vi "S4ICS Batch Processor.vi"() -> ()   [LabVIEW 2018]
uses:
  <vilib>/addons/zeromq/socket_type.ctl
  <vilib>/addons/zeromq/socket_options.ctl
  <vilib>/addons/zeromq/zmq_context.lvclass
  <vilib>/addons/zeromq/zeromq.lvlib
  <vilib>/addons/zeromq/zmq_socket.lvclass
panel:
  out "REQ":bool
  out "SUB":bool
  in  "batch file path":path
  in  "start":bool
  out "finish":bool
  in  "S4ICS REQ endpoint":string="tcp://192.168.1.170:54883"
  out "ASEL_RDY":bool
  out "GMIR_RDY":bool
  out "GFOC_RDY":bool
  out "CALW_RDY":bool
  out "WPSEL_RDY":bool
  out "WPROT_RDY":bool
  out "S4ICS PUB DATA":string
  out "PUB":bool
  in  "S4ICS PUB endpoint":string="tcp://192.168.1.170:54880"
  out "cmd #":i32
  out "current time":timestamp format="%<%H:%M:%S%3u\n%Y/%m/%d>T"
  out "batch cmd":string
  in  "allin":T1={"s4icsIP"="localhost", "s4icsPort"=54165, "mech name"="", "cmd"=[], "log"=refnum} {"s4icsPort" min=1025 step=1}
  in  "stop":bool
  # "S4ICS ZeroMQ Monitor and Batch Command Processor"
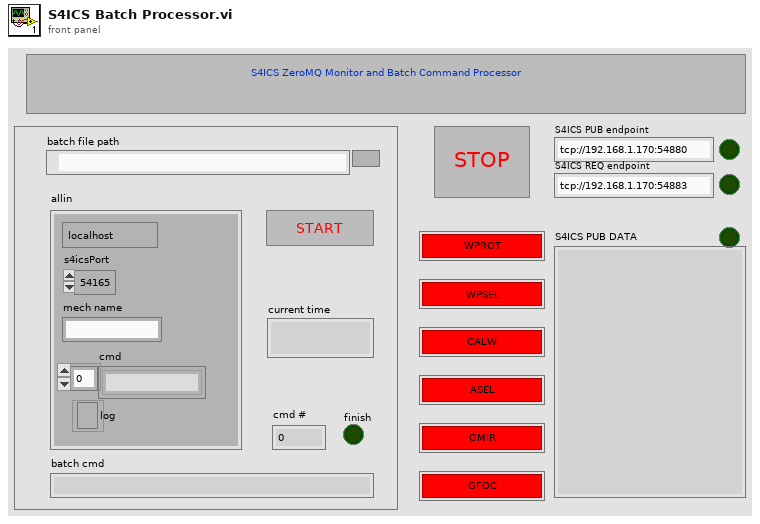
[diagram p1: front panel]
types:
  T1 = cluster{"s4icsIP":string, "s4icsPort":u16, "mech name":string, "cmd":string[], "log":refnum<file>}
  T2 = typedef "zeromq.lvlib/socket_type.ctl" = enum8{"ZMQ_PAIR", "ZMQ_PUB", "ZMQ_SUB", "ZMQ_REQ", "ZMQ_REP", "ZMQ_DEALER", "ZMQ_ROUTER", "ZMQ_PULL", "ZMQ_PUSH", "ZMQ_XPUB", "ZMQ_XSUB", "ZMQ_STREAM", "ZMQ_SERVER", "ZMQ_CLIENT", "ZMQ_RADIO", "ZMQ_DISH", "ZMQ_GATHER", "ZMQ_SCATTER", "ZMQ_DGRAM"}
  T3 = typedef "zeromq.lvlib/socket_options.ctl" = enum8{"NONE", "ZMQ_HWM", "<2>", "ZMQ_SWAP", "ZMQ_AFFINITY", "ZMQ_ROUTING_ID", "ZMQ_SUBSCRIBE", "ZMQ_UNSUBSCRIBE", "ZMQ_RATE", "ZMQ_RECOVERY_IVL", "ZMQ_MCAST_LOOP", "ZMQ_SNDBUF", "ZMQ_RCVBUF", "ZMQ_RCVMORE", "ZMQ_FD", "ZMQ_EVENTS", "ZMQ_TYPE", "ZMQ_LINGER", "ZMQ_RECONNECT_IVL", "ZMQ_BACKLOG", "ZMQ_RECOVERY_IVL_MSEC", "ZMQ_RECONNECT_IVL_MAX", "ZMQ_MAXMSGSIZE", "ZMQ_SNDHWM", "ZMQ_RCVHWM", "ZMQ_MULTICAST_HOPS", "<26>", "ZMQ_RCVTIMEO", "ZMQ_SNDTIMEO", "<29>", "<30>", "ZMQ_IPV4ONLY", "ZMQ_LAST_ENDPOINT", "ZMQ_ROUTER_MANDATORY", "ZMQ_TCP_KEEPALIVE", "ZMQ_TCP_KEEPALIVE_CNT", "ZMQ_TCP_KEEPALIVE_IDLE", "ZMQ_TCP_KEEPALIVE_INTVL", "ZMQ_TCP_ACCEPT_FILTER", "ZMQ_IMMEDIATE", "ZMQ_XPUB_VERBOSE", "ZMQ_ROUTER_RAW", "ZMQ_IPV6", "ZMQ_MECHANISM", "ZMQ_PLAIN_SERVER", "ZMQ_PLAIN_USERNAME", "ZMQ_PLAIN_PASSWORD", "ZMQ_CURVE_SERVER", "ZMQ_CURVE_PUBLICKEY", "ZMQ_CURVE_SECRETKEY", "ZMQ_CURVE_SERVERKEY", "ZMQ_PROBE_ROUTER", "ZMQ_REQ_CORRELATE", "ZMQ_REQ_RELAXED", "ZMQ_CONFLATE", "ZMQ_ZAP_DOMAIN", "ZMQ_ROUTER_HANDOVER", "ZMQ_TOS", "ZMQ_IPC_FILTER_PID", "ZMQ_IPC_FILTER_UID", "ZMQ_IPC_FILTER_GID", "ZMQ_CONNECT_ROUTING_ID", "ZMQ_GSSAPI_SERVER", "ZMQ_GSSAPI_PRINCIPAL", "ZMQ_GSSAPI_SERVICE_PRINCIPAL", "ZMQ_GSSAPI_PLAINTEXT", "ZMQ_HANDSHAKE_IVL", "<67>", "ZMQ_SOCKS_PROXY", "ZMQ_XPUB_NODROP", "ZMQ_BLOCKY", "ZMQ_XPUB_MANUAL", "ZMQ_XPUB_WELCOME_MSG", "ZMQ_STREAM_NOTIFY", "ZMQ_INVERT_MATCHING", "ZMQ_HEARTBEAT_IVL", "ZMQ_HEARTBEAT_TTL", "ZMQ_HEARTBEAT_TIMEOUT", "ZMQ_XPUB_VERBOSER", "ZMQ_CONNECT_TIMEOUT", "ZMQ_TCP_MAXRT", "ZMQ_THREAD_SAFE", "<82>", "<83>", "ZMQ_MULTICAST_MAXTPDU", "ZMQ_VMCI_BUFFER_SIZE", "ZMQ_VMCI_BUFFER_MIN_SIZE", "ZMQ_VMCI_BUFFER_MAX_SIZE", "ZMQ_VMCI_CONNECT_TIMEOUT", "ZMQ_USE_FD", "ZMQ_GSSAPI_PRINCIPAL_NAMETYPE", "ZMQ_GSSAPI_SERVICE_PRINCIPAL_NAMETYPE", "ZMQ_BINDTODEVICE", "ZMQ_ZAP_ENFORCE_DOMAIN", "ZMQ_LOOPBACK_FASTPATH", "ZMQ_METADATA", "ZMQ_MULTICAST_LOOP", "ZMQ_ROUTER_NOTIFY"}
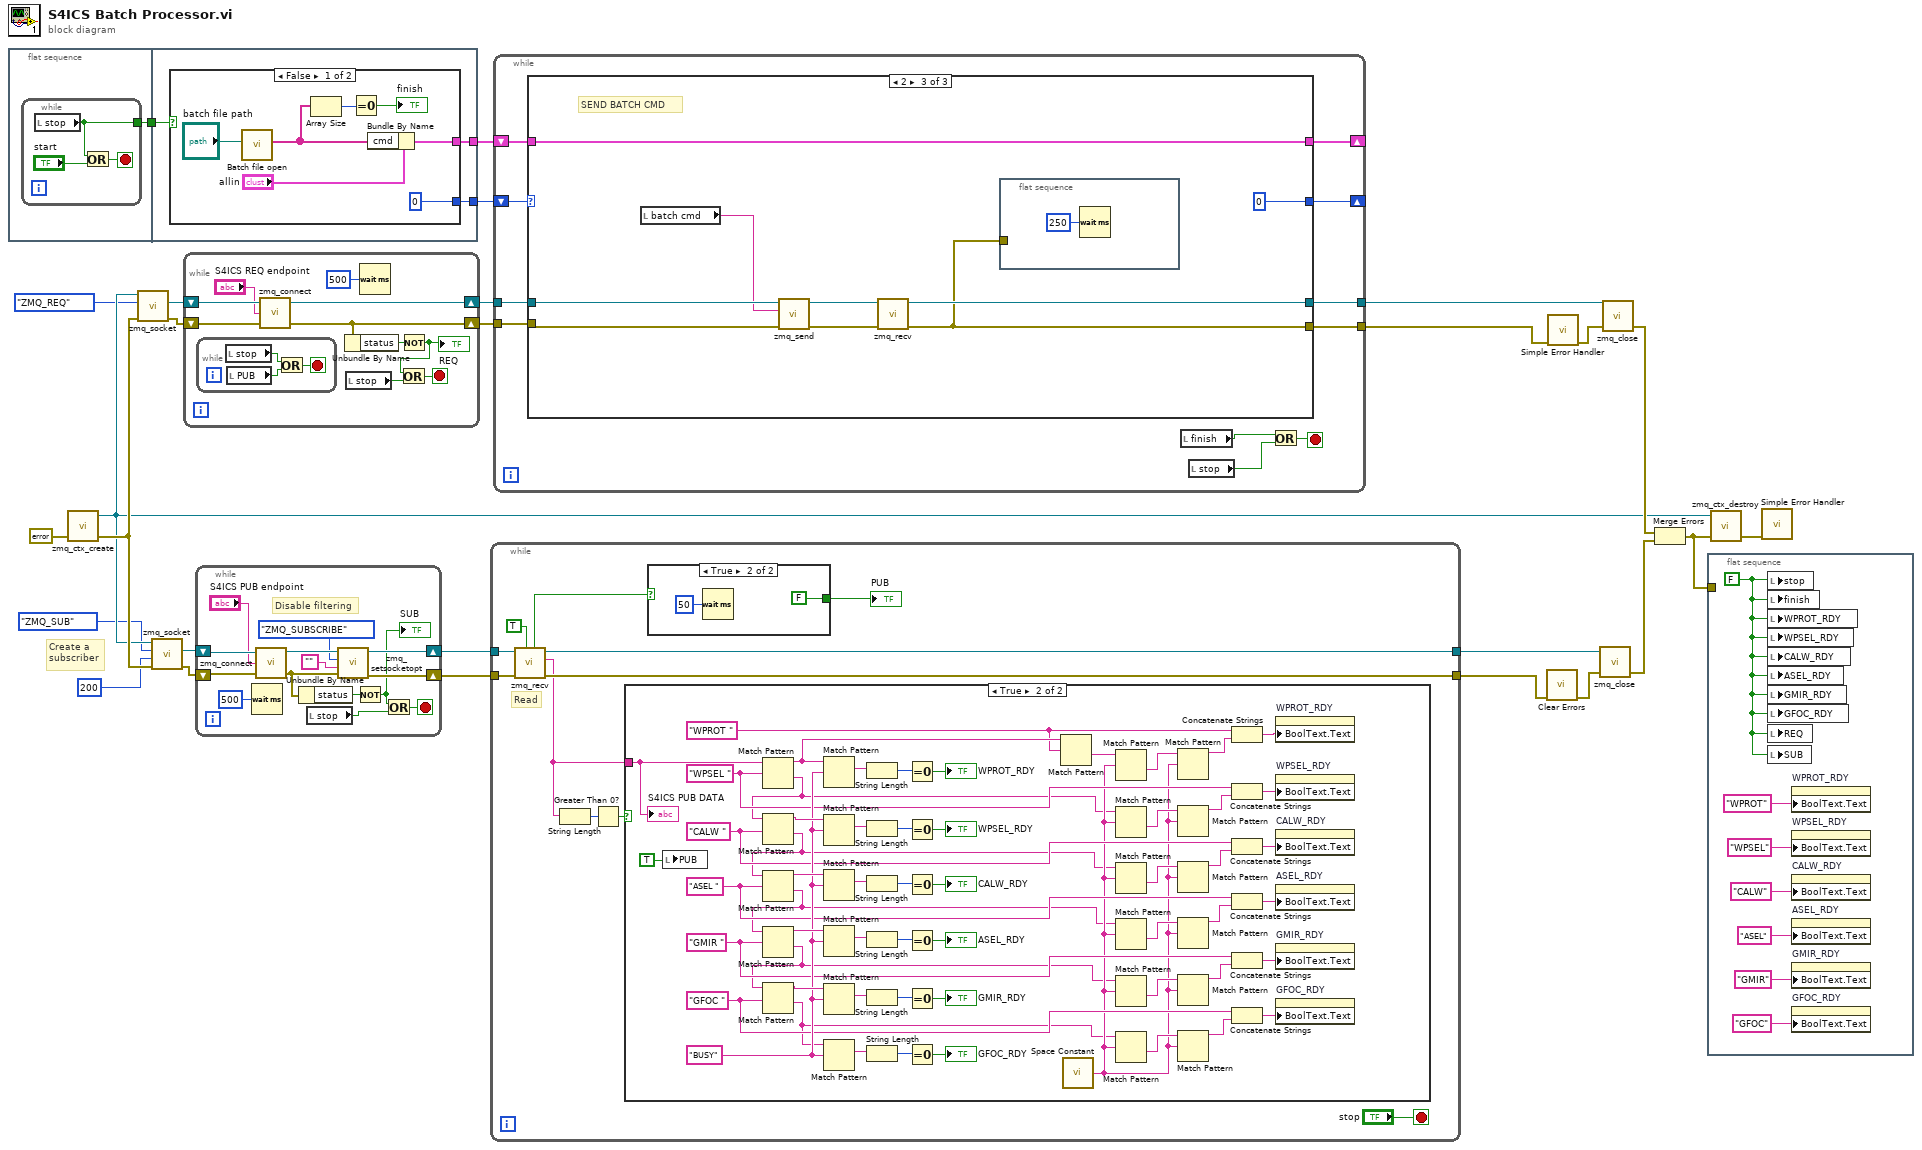
[diagram p0: block diagram]
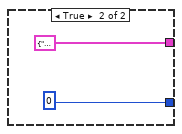
[diagram p2: hidden frame]
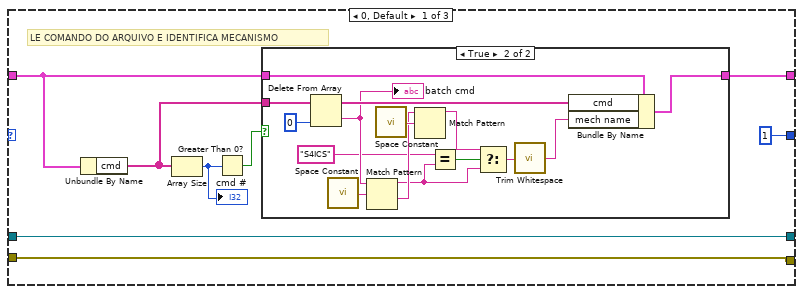
[diagram p3: hidden frame]
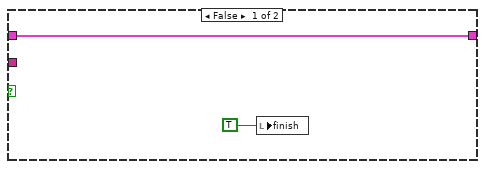
[diagram p4: hidden frame]
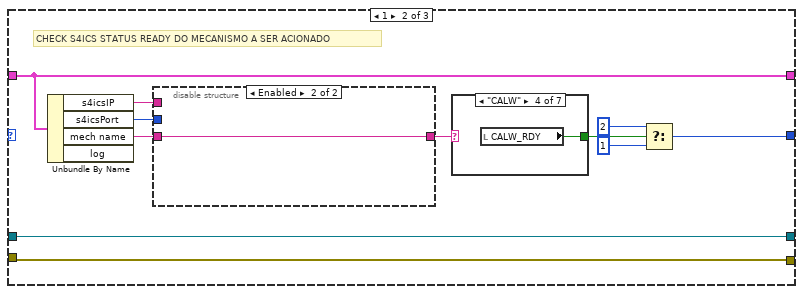
[diagram p5: hidden frame]
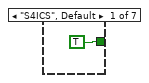
[diagram p6: hidden frame]
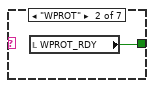
[diagram p7: hidden frame]
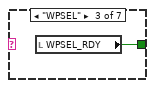
[diagram p8: hidden frame]
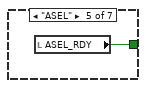
[diagram p9: hidden frame]
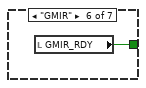
[diagram p10: hidden frame]
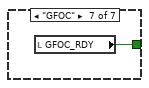
[diagram p11: hidden frame]
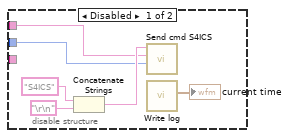
[diagram p12: hidden frame]
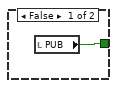
[diagram p14: hidden frame]
diagram:
  # "Create a \nsubscriber"
  n1 = flat-sequence {
    tunnel: [w28] -> w6
    tunnel: [w34] -> w16
    tunnel: [w33] -> w15
    tunnel: w6 -> [w32]
    frame #0 {
      n2 = while {
        tunnel: [w29] -> w28
        stop <- w30 stop-if-true
        n3 = local read "stop"() -> (w29:bool)
        n4 = Or(x=w29, y="start") -> (x .or. y?=w30:bool)
      }
    }
    frame #1 {
      n5 = case shown="False" w32 {
        tunnel: [u8 0 u8 0] -> w34
        tunnel: [w39 T1 {"s4icsIP"="", "s4icsPort"=0, "mech name"="", "cmd"=[], "log"=refnum} ("output cluster")] -> w33
        frame False {
          n6 = call "Batch file open.vi"("file path (use dialog)"="batch file path") -> ("cmd"=w38:string[])  [unwired: 10 in]
          n7 = Array Size(array=w38) -> (size(s)=w37:i32)
          n8 = Equal To 0?(x=w37) -> (x = 0?=→"finish":bool)
          n9 = Bundle By Name(cluster="allin", "cmd"=w38) -> (w39:T1)
        }
        frame True {
        }
      }
    }
  }
  n10 = call <vilib>:"zmq_ctx_create.vi"("error in"=errorcluster {"status"=FALSE, "code"=0, "source"=""}) -> ("error out"=w22:errorcluster, "context out"=w19:refnum<class "zmq_context.lvclass">)  [unwired: 3 in]
  n11 = call <vilib>:"zmq_socket.vi"("error in"=w22, "socket type"=socket_type."ZMQ_REQ", "context in"=w19) -> ("error out"=w14:errorcluster, "socket out"=w13:refnum<class "zmq_socket.lvclass">)  [unwired: 2 in, 1 out]
  n12 = call <vilib>:"zmq_socket.vi"("error in"=w22, "linger (ms)"=200, "socket type"=socket_type."ZMQ_SUB", "context in"=w19) -> ("error out"=w4:errorcluster, "socket out"=w3:refnum<class "zmq_socket.lvclass">)  [unwired: 1 in, 1 out]
  n13 = while {
    shift-right: [w49] -> w10
    shift-left: w14 -> [w53]
    shift-right: [w50] -> w11
    shift-left: w13 -> [w52]
    stop <- w46 stop-if-true
    n14 = while {
      stop <- w54 stop-if-true
      n15 = local read "stop"() -> (w55:bool)
      n16 = local read "PUB"() -> (w56:bool)
      n17 = Or(x=w55, y=w56) -> (x .or. y?=w54:bool)
    }
    n18 = call <vilib>:"zmq_connect.vi"("error in"=w53, "endpoint"="S4ICS REQ endpoint", "socket in"=w52) -> ("error out"=w49:errorcluster, "socket out"=w50:refnum<class "zmq_socket.lvclass">)  [unwired: 1 in]
    n19 = Unbundle By Name(w49) -> ("status"=w48:bool)
    n20 = local read "stop"() -> (w45:bool)
    n21 = Wait (ms)(milliseconds to wait=u32 500) -> ()  [unwired: 1 out]
    n22 = Not(x=w48) -> (.not. x?=w44:bool)
    "REQ" <- w44
    n23 = Or(x=w44, y=w45) -> (x .or. y?=w46:bool)
  }
  n24 = while {
    shift-right: [w70] -> w27
    shift-left: w4 -> [w68]
    shift-right: [w69] -> w26
    shift-left: w3 -> [w64]
    stop <- w59 stop-if-true
    # "Disable filtering"
    n25 = Wait (ms)(milliseconds to wait=u32 500) -> ()  [unwired: 1 out]
    n26 = call <vilib>:"zmq_connect.vi"("error in"=w68, "endpoint"="S4ICS PUB endpoint", "socket in"=w64) -> ("error out"=w60:errorcluster, "socket out"=w67:refnum<class "zmq_socket.lvclass">)  [unwired: 1 in]
    n27 = Unbundle By Name(w60) -> ("status"=w61:bool)
    n28 = local read "stop"() -> (w62:bool)
    n29 = call <vilib>:"zmq_setsocketopt.vi"("error in"=w60, "value"="", "option"=socket_options."ZMQ_SUBSCRIBE", "socket in"=w67) -> ("error out"=w70:errorcluster, "socket out"=w69:refnum<class "zmq_socket.lvclass">)  [unwired: 2 in]
    n30 = Not(x=w61) -> (.not. x?=w57:bool)
    "SUB" <- w57
    n31 = Or(x=w57, y=w62) -> (x .or. y?=w59:bool)
  }
  n32 = while {
    tunnel: w27 -> [w79]
    tunnel: w26 -> [w80]
    tunnel: [w76] -> w23
    tunnel: [w75] -> w25
    stop <- "stop" stop-if-true
    # "Read"
    n33 = call <vilib>:"zmq_recv.vi"("no block? (F)"=TRUE, "error in"=w79, "socket in"=w80) -> ("error out"=w75:errorcluster, "data"=w72:string, "socket out"=w76:refnum<class "zmq_socket.lvclass">, "timeout?"=w78:bool)  [unwired: 2 in, 1 out]
    n34 = String Length(string=w72) -> (length=w74:i32)
    n35 = Greater Than 0?(x=w74) -> (x > 0?=w73:bool)
    n36 = case shown="True" w73 {
      tunnel: w72 -> [_ w137]
      frame False {
      }
      frame True {
        w111 = "WPROT " ("regular expression")
        w106 = "GFOC " ("regular expression")
        w107 = "GMIR " ("regular expression")
        w109 = "CALW " ("regular expression")
        w114 = "BUSY" ("regular expression")
        w110 = "WPSEL " ("regular expression")
        w108 = "ASEL " ("regular expression")
        n37 = local write "PUB"(TRUE) -> ()
        n38 = Match Pattern(string=w137, regular expression=w110) -> (before substring=w113:string, after substring=w86:string)  [unwired: 1 in, 2 out]
        n39 = Match Pattern(string=w86, regular expression=w109) -> (before substring=w130:string, after substring=w85:string)  [unwired: 1 in, 2 out]
        n40 = Match Pattern(string=w85, regular expression=w108) -> (before substring=w126:string, after substring=w84:string)  [unwired: 1 in, 2 out]
        n41 = Match Pattern(string=w84, regular expression=w107) -> (before substring=w115:string, after substring=w83:string)  [unwired: 1 in, 2 out]
        n42 = Match Pattern(string=w83, regular expression=w106) -> (before substring=w122:string, after substring=w82:string)  [unwired: 1 in, 2 out]
        n43 = Match Pattern(string=w113, regular expression=w114) -> (match substring=w136:string)  [unwired: 1 in, 3 out]
        n44 = Match Pattern(string=w130, regular expression=w114) -> (match substring=w131:string)  [unwired: 1 in, 3 out]
        n45 = Match Pattern(string=w126, regular expression=w114) -> (match substring=w129:string)  [unwired: 1 in, 3 out]
        n46 = Match Pattern(string=w115, regular expression=w114) -> (match substring=w116:string)  [unwired: 1 in, 3 out]
        n47 = Match Pattern(string=w122, regular expression=w114) -> (match substring=w121:string)  [unwired: 1 in, 3 out]
        n48 = Match Pattern(string=w82, regular expression=w114) -> (match substring=w123:string)  [unwired: 1 in, 3 out]
        n49 = String Length(string=w136) -> (length=w135:i32)
        n50 = String Length(string=w131) -> (length=w132:i32)
        n51 = String Length(string=w129) -> (length=w128:i32)
        n52 = String Length(string=w116) -> (length=w117:i32)
        n53 = String Length(string=w121) -> (length=w120:i32)
        n54 = String Length(string=w123) -> (length=w124:i32)
        n55 = Equal To 0?(x=w135) -> (x = 0?=→"WPROT_RDY":bool)
        n56 = Equal To 0?(x=w132) -> (x = 0?=→"WPSEL_RDY":bool)
        n57 = Equal To 0?(x=w128) -> (x = 0?=→"CALW_RDY":bool)
        n58 = Equal To 0?(x=w117) -> (x = 0?=→"ASEL_RDY":bool)
        n59 = Equal To 0?(x=w120) -> (x = 0?=→"GMIR_RDY":bool)
        n60 = Equal To 0?(x=w124) -> (x = 0?=→"GFOC_RDY":bool)
        n61 = Match Pattern(string=w113, regular expression=w111) -> (after substring=w112:string)  [unwired: 1 in, 3 out]
        n62 = call <vilib>:"Space Constant.vi"() -> ("String"=w87:string)
        n63 = Match Pattern(string=w112, regular expression=w87) -> (after substring=w99:string)  [unwired: 1 in, 3 out]
        n64 = Match Pattern(string=w86, regular expression=w87) -> (after substring=w97:string)  [unwired: 1 in, 3 out]
        n65 = Match Pattern(string=w85, regular expression=w87) -> (after substring=w91:string)  [unwired: 1 in, 3 out]
        n66 = Match Pattern(string=w84, regular expression=w87) -> (after substring=w90:string)  [unwired: 1 in, 3 out]
        n67 = Match Pattern(string=w83, regular expression=w87) -> (after substring=w89:string)  [unwired: 1 in, 3 out]
        n68 = Match Pattern(string=w82, regular expression=w87) -> (after substring=w88:string)  [unwired: 1 in, 3 out]
        n69 = Match Pattern(string=w99, regular expression=w87) -> (before substring=w98:string)  [unwired: 1 in, 3 out]
        n70 = Match Pattern(string=w97, regular expression=w87) -> (before substring=w96:string)  [unwired: 1 in, 3 out]
        n71 = Match Pattern(string=w91, regular expression=w87) -> (before substring=w95:string)  [unwired: 1 in, 3 out]
        n72 = Match Pattern(string=w90, regular expression=w87) -> (before substring=w94:string)  [unwired: 1 in, 3 out]
        n73 = Match Pattern(string=w89, regular expression=w87) -> (before substring=w93:string)  [unwired: 1 in, 3 out]
        n74 = Match Pattern(string=w88, regular expression=w87) -> (before substring=w92:string)  [unwired: 1 in, 3 out]
        n75 = Concatenate Strings(w111, w98) -> (w100:string)
        n76 = Concatenate Strings(w110, w96) -> (w101:string)
        n77 = Concatenate Strings(w109, w95) -> (w102:string)
        n78 = Concatenate Strings(w108, w94) -> (w103:string)
        n79 = Concatenate Strings(w107, w93) -> (w104:string)
        n80 = Concatenate Strings(w106, w92) -> (w105:string)
        n81 = property on="WPROT_RDY" class="Bool (strict)"("BoolText.Text"=w100) -> ()  [unwired: 2 in, 2 out]
        n82 = property on="WPSEL_RDY" class="Bool (strict)"("BoolText.Text"=w101) -> ()  [unwired: 2 in, 2 out]
        n83 = property on="CALW_RDY" class="Bool (strict)"("BoolText.Text"=w102) -> ()  [unwired: 2 in, 2 out]
        n84 = property on="ASEL_RDY" class="Bool (strict)"("BoolText.Text"=w103) -> ()  [unwired: 2 in, 2 out]
        n85 = property on="GMIR_RDY" class="Bool (strict)"("BoolText.Text"=w104) -> ()  [unwired: 2 in, 2 out]
        n86 = property on="GFOC_RDY" class="Bool (strict)"("BoolText.Text"=w105) -> ()  [unwired: 2 in, 2 out]
        "S4ICS PUB DATA" <- w137
      }
    }
    n87 = case shown="True" w78 {
      tunnel: [w139 FALSE] -> w77
      frame False {
        n88 = local read "PUB"() -> (w139:bool)
      }
      frame True {
        n89 = Wait (ms)(milliseconds to wait=u32 50) -> ()  [unwired: 1 out]
      }
    }
    "PUB" <- w77
  }
  n90 = while {
    shift-right: [w151] -> _
    shift-left: w16 -> [w152]
    shift-right: [w149] -> _
    shift-left: w15 -> [w150]
    tunnel: w11 -> [w148]
    tunnel: w10 -> [w147]
    tunnel: [w146] -> w9
    tunnel: [w145] -> w8
    stop <- w142 stop-if-true
    n91 = case shown="2" w152 {
      tunnel: [u8 1 ("x+1") w186 u8 0 ("x+1")] -> w151
      tunnel: w150 -> [w158 w188 w211]
      tunnel: [w156 w188 w211] -> w149
      tunnel: w148 -> [w154 w179 w207]
      tunnel: w147 -> [w153 w178 w206]
      tunnel: [w154 w179 w204] -> w146
      tunnel: [w153 w178 w203] -> w145
      frame 0, Default {
        # "LE COMANDO DO ARQUIVO E IDENTIFICA MECANISMO"
        n92 = Unbundle By Name(w158) -> ("cmd"=w155:string[])
        n93 = Array Size(array=w155) -> (size(s)=w160:i32)
        "cmd #" <- w160
        n94 = Greater Than 0?(x=w160) -> (x > 0?=w159:bool)
        n95 = case shown="True" w159 {
          tunnel: w155 -> [_ w177]
          tunnel: w158 -> [w162 w176]
          tunnel: [w162 w175] -> w156
          frame False {
            n96 = local write "finish"(TRUE) -> ()
          }
          frame True {
            n97 = Delete From Array(array=w177, index=0) -> (deleted portion=w171:string, array with subset deleted=w174:string[])  [unwired: 1 in]
            "batch cmd" <- w171
            n98 = call <vilib>:"Space Constant.vi"() -> ("String"=w172:string)
            n99 = Match Pattern(string=w171, regular expression=w172) -> (before substring=w165:string, after substring=w169:string)  [unwired: 1 in, 2 out]
            n100 = call <vilib>:"Space Constant.vi"() -> ("String"=w170:string)
            n101 = Match Pattern(string=w169, regular expression=w170) -> (before substring=w166:string)  [unwired: 1 in, 3 out]
            n102 = Equal?(x="S4ICS", y=w165) -> (x = y?=w167:bool)
            n103 = Select(t=w166, s=w167, f=w165) -> (s? t:f=w164:string)
            n104 = call <vilib>:"Trim Whitespace.vi"("string"=w164) -> ("trimmed string"=w163:string)  [unwired: 1 in]
            n105 = Bundle By Name(cluster=w176, "cmd"=w174, "mech name"=w163) -> (w175:T1)
          }
        }
      }
      frame 1 {
        # "CHECK S4ICS STATUS READY DO MECANISMO A SER ACIONADO"
        n106 = Unbundle By Name(w188) -> ("s4icsIP"=w183:string, "s4icsPort"=w182:u16, "mech name"=w181:string)  [unwired: 1 out]
        n107 = disable-structure shown="Enabled" {
          disable-tunnel: w183 -> [w197 _]
          disable-tunnel: w182 -> [w196 _]
          disable-tunnel: w181 -> [_ w202]
          disable-tunnel: [_ w202] -> w180
          frame Disabled {
            n108 = Concatenate Strings("S4ICS", "\r\n") -> (w199:string)
            n109 = call "Send cmd S4ICS.vi"("port"=w196, "address"=w197, "data in"=w199) -> ()  [unwired: 7 in, 2 out]
            n110 = call "Write log.vi"() -> ("current time"=→"current time":timestamp)  [unwired: 10 in, 1 out]
          }
          frame Enabled {
          }
        }
        n111 = case shown="\"CALW\"" w180 {
          tunnel: [TRUE w190 w191 w192 w193 w194 w195] -> w187
          frame "S4ICS", Default {
          }
          frame "WPROT" {
            n112 = local read "WPROT_RDY"() -> (w190:bool)
          }
          frame "WPSEL" {
            n113 = local read "WPSEL_RDY"() -> (w191:bool)
          }
          frame "CALW" {
            n114 = local read "CALW_RDY"() -> (w192:bool)
          }
          frame "ASEL" {
            n115 = local read "ASEL_RDY"() -> (w193:bool)
          }
          frame "GMIR" {
            n116 = local read "GMIR_RDY"() -> (w194:bool)
          }
          frame "GFOC" {
            n117 = local read "GFOC_RDY"() -> (w195:bool)
          }
        }
        n118 = Select(t=u8 2 ("f"), s=w187, f=u8 1) -> (s? t:f=w186:u8)
      }
      frame 2 {
        # "SEND BATCH CMD"
        n119 = local read "batch cmd"() -> (w205:string)
        n120 = call <vilib>:"zmq_send.vi"("error in"=w206, "data"=w205, "socket in"=w207) -> ("error out"=w208:errorcluster, "socket out"=w209:refnum<class "zmq_socket.lvclass">)  [unwired: 4 in]
        n121 = call <vilib>:"zmq_recv.vi"("error in"=w208, "socket in"=w209) -> ("error out"=w203:errorcluster, "socket out"=w204:refnum<class "zmq_socket.lvclass">)  [unwired: 3 in, 3 out]
        n122 = flat-sequence {
          tunnel: w203 -> [_]
          frame #0 {
            n123 = Wait (ms)(milliseconds to wait=u32 250) -> ()  [unwired: 1 out]
          }
        }
      }
    }
    n124 = local read "finish"() -> (w143:bool)
    n125 = local read "stop"() -> (w144:bool)
    n126 = Or(x=w143, y=w144) -> (x .or. y?=w142:bool)
  }
  n127 = call <vilib>:"Clear Errors.vi"("error in (no error)"=w25) -> ("error out"=w24:errorcluster)  [unwired: 5 in, 1 out]
  n128 = call <vilib>:"Simple Error Handler.vi"("error in (no error)"=w8) -> ("error out"=w7:errorcluster)  [unwired: 4 in, 4 out]
  n129 = call <vilib>:"zmq_close.vi"("error in"=w24, "socket"=w23) -> ("error out"=w20:errorcluster)  [unwired: 3 in]
  n130 = call <vilib>:"zmq_close.vi"("error in"=w7, "socket"=w9) -> ("error out"=w21:errorcluster)  [unwired: 3 in]
  n131 = Merge Errors(w21, w20) -> (w17:errorcluster)
  n132 = flat-sequence {
    tunnel: w17 -> [_]
    frame #0 {
      w213 = FALSE
      n133 = local write "stop"(w213) -> ()
      n134 = local write "finish"(w213) -> ()
      n135 = local write "WPROT_RDY"(w213) -> ()
      n136 = local write "WPSEL_RDY"(w213) -> ()
      n137 = local write "CALW_RDY"(w213) -> ()
      n138 = local write "ASEL_RDY"(w213) -> ()
      n139 = local write "GMIR_RDY"(w213) -> ()
      n140 = local write "GFOC_RDY"(w213) -> ()
      n141 = local write "REQ"(w213) -> ()
      n142 = local write "SUB"(w213) -> ()
      n143 = property on="WPROT_RDY" class="Bool (strict)"("BoolText.Text"="WPROT" ("regular expression")) -> ()  [unwired: 2 in, 2 out]
      n144 = property on="WPSEL_RDY" class="Bool (strict)"("BoolText.Text"="WPSEL" ("regular expression")) -> ()  [unwired: 2 in, 2 out]
      n145 = property on="CALW_RDY" class="Bool (strict)"("BoolText.Text"="CALW" ("regular expression")) -> ()  [unwired: 2 in, 2 out]
      n146 = property on="ASEL_RDY" class="Bool (strict)"("BoolText.Text"="ASEL" ("regular expression")) -> ()  [unwired: 2 in, 2 out]
      n147 = property on="GMIR_RDY" class="Bool (strict)"("BoolText.Text"="GMIR" ("regular expression")) -> ()  [unwired: 2 in, 2 out]
      n148 = property on="GFOC_RDY" class="Bool (strict)"("BoolText.Text"="GFOC" ("regular expression")) -> ()  [unwired: 2 in, 2 out]
    }
  }
  n149 = call <vilib>:"zmq_ctx_destroy.vi"("error in"=w17, "context in"=w19) -> ("error out"=w18:errorcluster)  [unwired: 3 in]
  n150 = call <vilib>:"Simple Error Handler.vi"("error in (no error)"=w18) -> ()  [unwired: 4 in, 5 out]
